vi "matscript.vi"() -> ()   [LabVIEW 2021]
panel:
  out "w4":dbl
  out "w3":dbl
  out "w2":dbl
  out "w1":dbl
  in  "k":dbl
  in  "phi2":dbl
  in  "phi1":dbl
  in  "phi":dbl
  in  "deltat":dbl
  in  "f":dbl
  in  "A":dbl
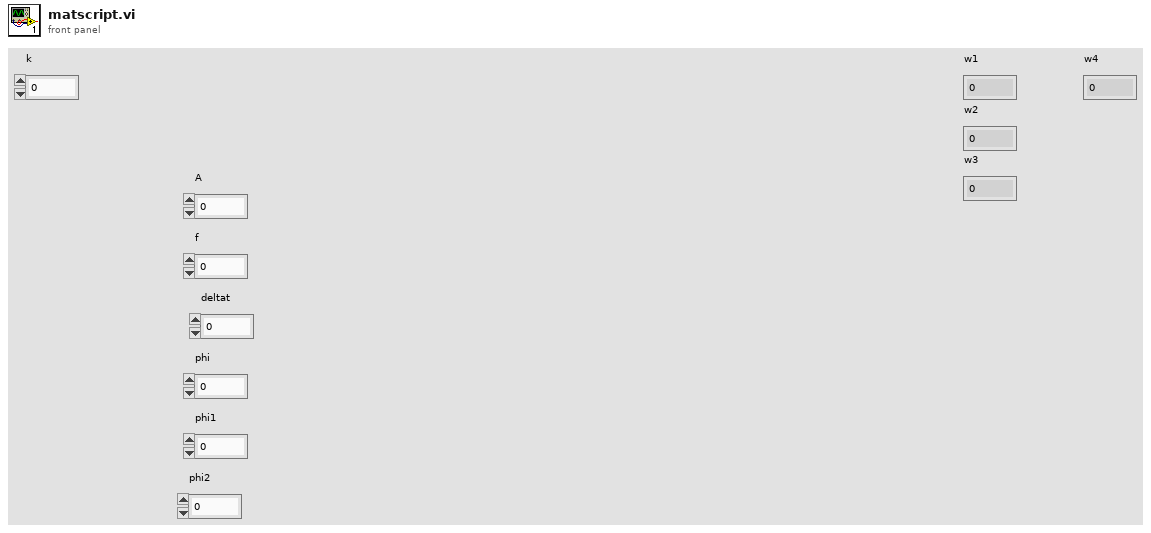
[diagram p1: front panel]
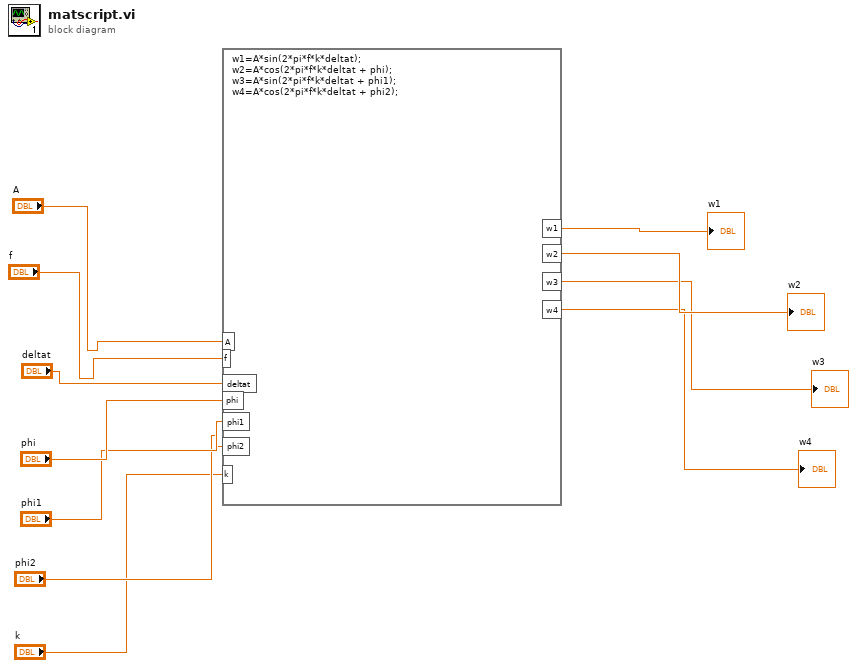
[diagram p0: block diagram]
diagram:
  n1 = formula code="w1=A*sin(2*pi*f*k*deltat);\nw2=A*cos(2*pi*f*k*deltat + phi);\nw3=A*sin(2*pi*f*k*deltat + phi1);\nw4=A*cos(2*pi*f*k*deltat + phi2);"("A"="A", "f"="f", "deltat"="deltat", "phi"="phi", "phi1"="phi1", "phi2"="phi2", "k"="k") -> ("w1"=→"w1":dbl, "w2"=→"w2":dbl, "w3"=→"w3":dbl, "w4"=→"w4":dbl)
